vi "getInheritanceChain.vi"(8 "error in (no error)":errorcluster, 11 "DataObj in":refnum<class "DataObj.lvclass">) -> (0 "error out":errorcluster, 2 "Inheritance Chain":string[](array[string]), 3 "DataObj out":refnum<class "DataObj.lvclass">)   [LabVIEW 2009, in "DataObj.lvclass"]
doc: "Returns the inheritance chain."
uses:
  DataObj.lvclass
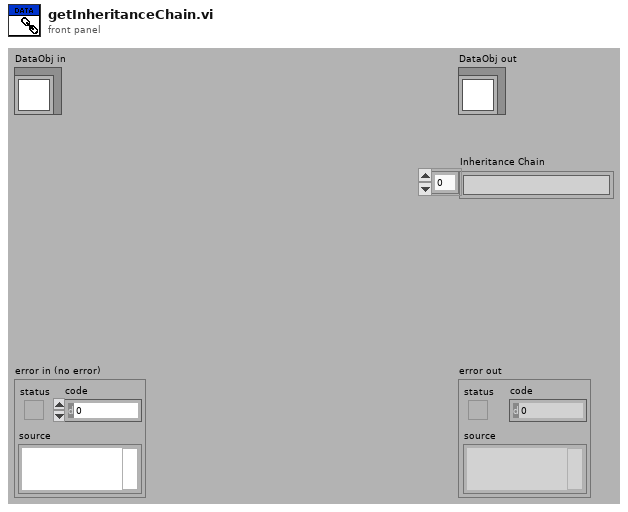
[diagram p1: front panel]
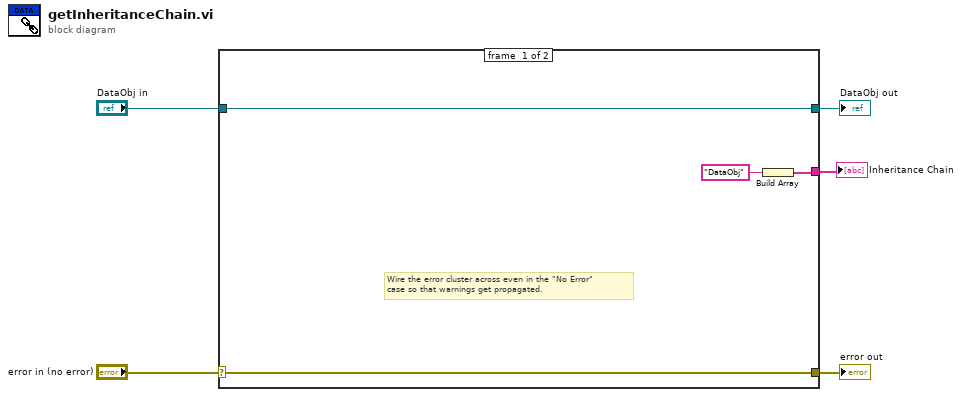
[diagram p0: block diagram]
diagram:
  n1 = case shown="No Error" "error in (no error)" {
    selector: "error in (no error)" -> [w8 w11]
    tunnel: [w8 w11] -> w4
    tunnel: [w9 w10] -> w2
    tunnel: "DataObj in" -> [w9 w10]
    tunnel: [w7 _] -> w1
    frame #0 {
      # "Wire the error cluster across even in the \"No Error\"\ncase so that warnings get propagated."
      n2 = Build Array("DataObj") -> (w7:string[])
    }
    frame #1 {
    }
  }
  "error out" <- w4
  "DataObj out" <- w2
  "Inheritance Chain" <- w1
